vi "set laser delays.vi"(8 "error in (no error)":errorcluster, 10 "offdelay":i16, 11 "ondelay":i16) -> (0 "error out":errorcluster)   [LabVIEW 2015, in "SCANalone4x64.lvlib"]
doc: "__declspec(dllimport) void __stdcall set_laser_delays(short ondelay, short offdelay);"
uses:
  <userlib>/SCANalone4x64/SCANalone4x64.lvlib
  <userlib>/SCANalone4x64/SCANalone4x64.dll
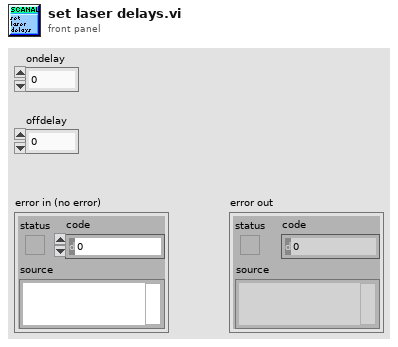
[diagram p1: front panel]
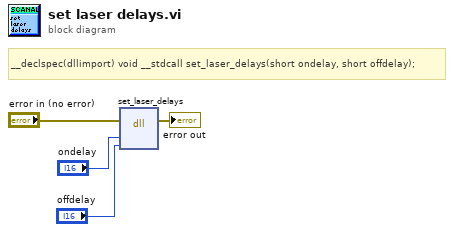
[diagram p0: block diagram]
diagram:
  # "__declspec(dllimport) void __stdcall set_laser_delays(short ondelay, short offdelay);"
  n1 = dll-call lib="C:/Program Files/National Instruments/LabVIEW 2015/user.lib/SCANalone4x64/SCANalone4x64.*" fn="set_laser_delays"(error in="error in (no error)", "ondelay"="ondelay", "offdelay"="offdelay") -> (error out=→"error out":errorcluster)  [unwired: 5 in, 1 out]
